vi "AddParamChannels_Insert SDI SSM Parity.vi"(8 "error in (no error)":errorcluster, 9 "Label Name":string, 11 "Label Parameters":T2) -> (0 "error out":errorcluster, 3 "Parameters Out":T1[](array[typedef]))   [LabVIEW 2020, in "Ballard Arinc-429 System Explorer.lvlib"]
uses:
  Ballard Arinc-429 System Explorer.lvlib
  Parse Parameters File/XML_Label.ctl
  Parse Parameters File/XML_Parameter.ctl
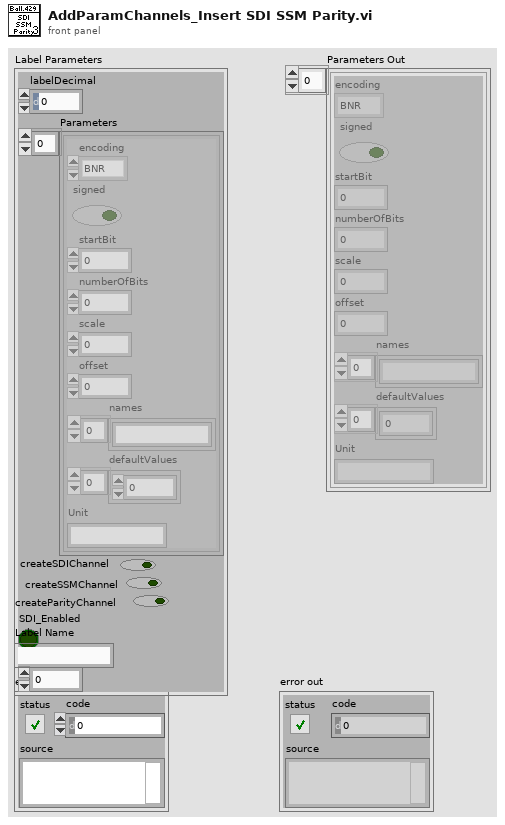
[diagram p1: front panel]
types:
  T1 = typedef "XML_Parameter.ctl" = cluster{"encoding":enum16{"BNR", "BCD", "Discrete"}, "signed":bool, "startBit":i32, "numberOfBits":i32, "scale":dbl, "offset":dbl, "names":string[], "defaultValues":dbl[], "Unit":string}
  T2 = typedef "XML_Label.ctl" = cluster{"labelDecimal":i32, "Parameters":T1[], "createSDIChannel":bool, "createSSMChannel":bool, "createParityChannel":bool, "SDI_Enabled":bool, "SDIValue":u8}
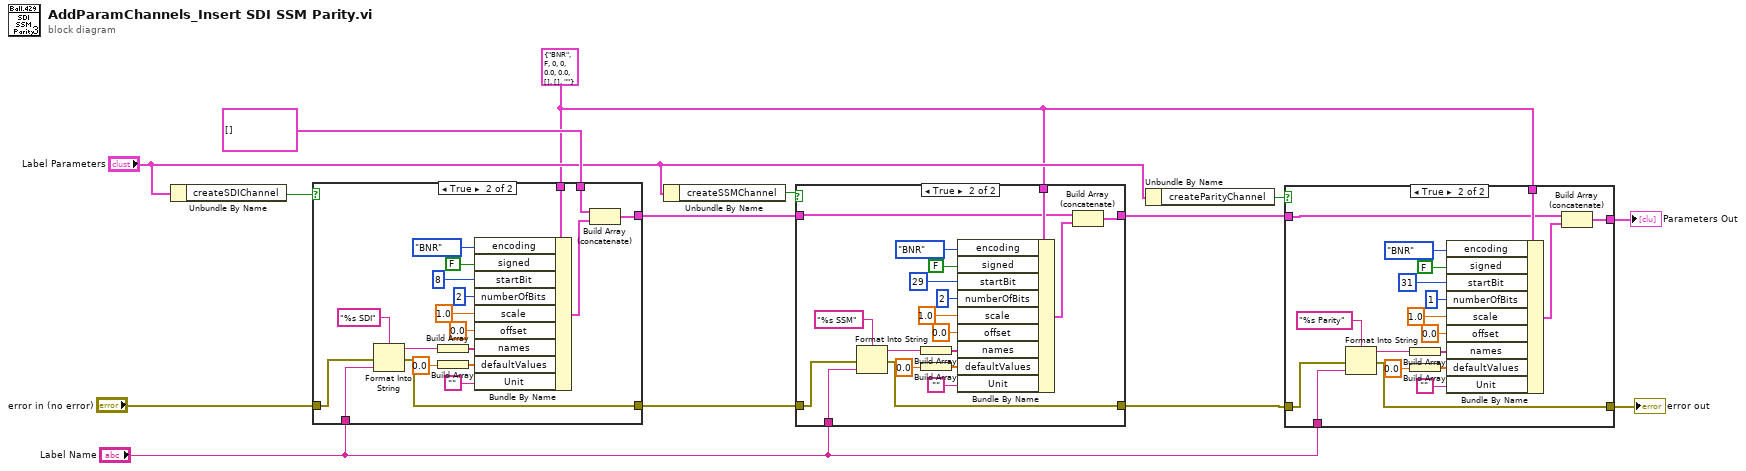
[diagram p0: block diagram]
diagram:
  w2 = T1 {"encoding"=enum."BNR", "signed"=FALSE, "startBit"=0, "numberOfBits"=0, "scale"=0.0, "offset"=0.0, "names"=[], "defaultValues"=[], "Unit"=""} ("Parameter")
  n1 = Unbundle By Name("Label Parameters") -> ("createSDIChannel"=w14:bool)
  n2 = case shown="True" w14 {
    tunnel: w2 -> [_ w35]
    tunnel: T1[] [] -> [w16 w25]
    tunnel: [w16 w23] -> w10
    tunnel: "Label Name" -> [_ w22]
    tunnel: "error in (no error)" -> [w15 w18]
    tunnel: [w15 w17] -> w9
    frame False {
    }
    frame True {
      n3 = Format Into String(format string="%s SDI", error in=w18, w22) -> (resulting string=w21:string, error out=w17:errorcluster)  [unwired: 1 in]
      n4 = Build Array(w21) -> (w20:string[])
      n5 = Build Array(0.0 ("offset")) -> (w27:dbl[])
      n6 = Bundle By Name(cluster=w35, "encoding"=enum16{"BNR", "BCD", "Discrete"}."BNR", "signed"=FALSE, "startBit"=8, "numberOfBits"=2, "scale"=1.0, "offset"=0.0, "names"=w20, "defaultValues"=w27, "Unit"="") -> (w24:T1)
      n7 = Build Array (concatenate)(w25, w24) -> (w23:T1[])
    }
  }
  n8 = Unbundle By Name("Label Parameters") -> ("createSSMChannel"=w11:bool)
  n9 = case shown="True" w11 {
    tunnel: [w36 w46] -> w3
    tunnel: "Label Name" -> [_ w45]
    tunnel: w9 -> [w37 w41]
    tunnel: [w37 w40] -> w6
    tunnel: w10 -> [w36 w38]
    tunnel: w2 -> [_ w39]
    frame False {
    }
    frame True {
      n10 = Format Into String(format string="%s SSM", error in=w41, w45) -> (resulting string=w44:string, error out=w40:errorcluster)  [unwired: 1 in]
      n11 = Build Array(w44) -> (w43:string[])
      n12 = Build Array(0.0 ("offset")) -> (w49:dbl[])
      n13 = Bundle By Name(cluster=w39, "encoding"=enum16{"BNR", "BCD", "Discrete"}."BNR", "signed"=FALSE, "startBit"=29, "numberOfBits"=2, "scale"=1.0, "offset"=0.0, "names"=w43, "defaultValues"=w49, "Unit"="") -> (w47:T1)
      n14 = Build Array (concatenate)(w38, w47) -> (w46:T1[])
    }
  }
  n15 = Unbundle By Name("Label Parameters") -> ("createParityChannel"=w7:bool)
  n16 = case shown="True" w7 {
    tunnel: "Label Name" -> [_ w67]
    tunnel: w6 -> [w58 w63]
    tunnel: [w58 w62] -> w4
    tunnel: w3 -> [w57 w60]
    tunnel: w2 -> [_ w61]
    tunnel: [w57 w59] -> w1
    frame False {
    }
    frame True {
      n17 = Format Into String(format string="%s Parity", error in=w63, w67) -> (resulting string=w66:string, error out=w62:errorcluster)  [unwired: 1 in]
      n18 = Build Array(w66) -> (w65:string[])
      n19 = Build Array(0.0 ("offset")) -> (w70:dbl[])
      n20 = Bundle By Name(cluster=w61, "encoding"=enum16{"BNR", "BCD", "Discrete"}."BNR", "signed"=FALSE, "startBit"=31, "numberOfBits"=1, "scale"=1.0, "offset"=0.0, "names"=w65, "defaultValues"=w70, "Unit"="") -> (w68:T1)
      n21 = Build Array (concatenate)(w60, w68) -> (w59:T1[])
    }
  }
  "error out" <- w4
  "Parameters Out" <- w1
